vi "Font Style.vi"(2 "error in (no error)":errorcluster, 3 "Font Settings":T2={"Charset (-1)"=-1, "Weight (-1)"=-1, "Name"="", "Size"=" "}, 4 "Text Options":T1, 5 "NIReports.Report":refnum<k7>) -> (0 "error out":errorcluster, 1 "NIReports.Report out":refnum<k7>)   [LabVIEW 2015, in "NI_ReportGenerationCore.lvlib"]
uses:
  <vilib>/Utility/NIReport.llb/NI_ReportGenerationCore.lvlib
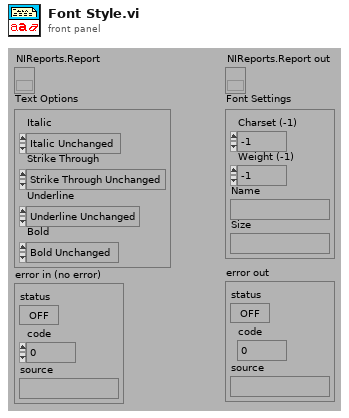
[diagram p1: front panel]
types:
  T1 = cluster{"Italic":enum16{"Italic Unchanged", "Italic On", "Italic Off"}, "Strike Through":enum16{"Strike Through Unchanged", "Strike Through On", "Strike Through Off"}, "Underline":enum16{"Underline Unchanged", "Underline On", "Underline Off"}, "Bold":enum16{"Bold Unchanged", "Bold On", "Bold Off"}}
  T2 = cluster{"Charset (-1)":i16, "Weight (-1)":i16, "Name":string, "Size":string}
  T3 = enum16{"Italic Unchanged", "Italic On", "Italic Off"}
  T4 = enum16{"Strike Through Unchanged", "Strike Through On", "Strike Through Off"}
  T5 = enum16{"Underline Unchanged", "Underline On", "Underline Off"}
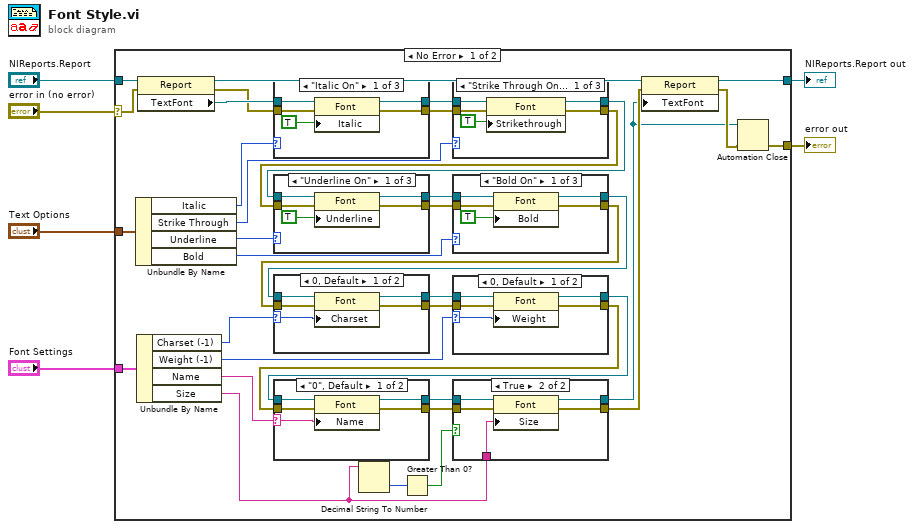
[diagram p0: block diagram]
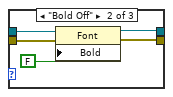
[diagram p6: hidden frame]
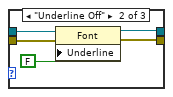
[diagram p8: hidden frame]
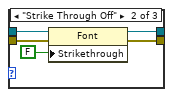
[diagram p10: hidden frame]
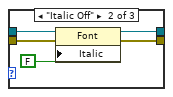
[diagram p12: hidden frame]
diagram:
  n1 = case shown="No Error" "error in (no error)" {
    selector: "error in (no error)" -> [w7 w119]
    tunnel: "Text Options" -> [w42 _]
    tunnel: "Font Settings" -> [w40 _]
    tunnel: "NIReports.Report" -> [w14 w120]
    tunnel: [w12 w120] -> w3
    tunnel: [w9 w119] -> w2
    frame No Error {
      n2 = Unbundle By Name(w42) -> ("Italic"=w41:T3, "Strike Through"=w35:T4, "Underline"=w32:T5, "Bold"=w29:enum16{"Bold Unchanged", "Bold On", "Bold Off"})
      n3 = Unbundle By Name(w40) -> ("Charset (-1)"=w28:i16, "Weight (-1)"=w23:i16, "Name"=w22:string, "Size"=w17:string)
      n4 = property class="Report"(reference=w14, error in=w7) -> (reference out=w13:refnum<k7>, error out=w38:errorcluster, "TextFont"=w39:refnum<k7>)
      n5 = case shown="\"Italic On\"" w41 {
        tunnel: w39 -> [w111 w115 w118]
        tunnel: w38 -> [w110 w114 w117]
        tunnel: [w108 w113 w118] -> w37
        tunnel: [w107 w112 w117] -> w36
        frame "Italic On" {
          n6 = property class="Font"(reference=w111, error in=w110, "Italic"=TRUE) -> (reference out=w108:refnum<k7>, error out=w107:errorcluster)
        }
        frame "Italic Off" {
          n7 = property class="Font"(reference=w115, error in=w114, "Italic"=FALSE) -> (reference out=w113:refnum<k7>, error out=w112:errorcluster)
        }
        frame "Italic Unchanged" {
        }
      }
      n8 = Decimal String To Number(string=w17) -> (number=w16:i32)  [unwired: 3 out]
      n9 = Greater Than 0?(x=w16) -> (x > 0?=w15:bool)
      n10 = case shown="\"Strike Through On\"" w35 {
        tunnel: w37 -> [w99 w103 w106]
        tunnel: w36 -> [w98 w102 w105]
        tunnel: [w96 w101 w106] -> w34
        tunnel: [w95 w100 w105] -> w33
        frame "Strike Through On" {
          n11 = property class="Font"(reference=w99, error in=w98, "Strikethrough"=TRUE ("Italic")) -> (reference out=w96:refnum<k7>, error out=w95:errorcluster)
        }
        frame "Strike Through Off" {
          n12 = property class="Font"(reference=w103, error in=w102, "Strikethrough"=FALSE ("Italic")) -> (reference out=w101:refnum<k7>, error out=w100:errorcluster)
        }
        frame "Strike Through Unchanged" {
        }
      }
      n13 = case shown="\"Underline On\"" w32 {
        tunnel: w34 -> [w87 w91 w94]
        tunnel: w33 -> [w86 w90 w93]
        tunnel: [w84 w89 w94] -> w30
        tunnel: [w83 w88 w93] -> w31
        frame "Underline On" {
          n14 = property class="Font"(reference=w87, error in=w86, "Underline"=TRUE ("Italic")) -> (reference out=w84:refnum<k7>, error out=w83:errorcluster)
        }
        frame "Underline Off" {
          n15 = property class="Font"(reference=w91, error in=w90, "Underline"=FALSE ("Italic")) -> (reference out=w89:refnum<k7>, error out=w88:errorcluster)
        }
        frame "Underline Unchanged" {
        }
      }
      n16 = case shown="\"Bold On\"" w29 {
        tunnel: w30 -> [w75 w79 w82]
        tunnel: w31 -> [w74 w78 w81]
        tunnel: [w72 w77 w82] -> w27
        tunnel: [w71 w76 w81] -> w26
        frame "Bold On" {
          n17 = property class="Font"(reference=w75, error in=w74, "Bold"=TRUE ("Italic")) -> (reference out=w72:refnum<k7>, error out=w71:errorcluster)
        }
        frame "Bold Off" {
          n18 = property class="Font"(reference=w79, error in=w78, "Bold"=FALSE ("Italic")) -> (reference out=w77:refnum<k7>, error out=w76:errorcluster)
        }
        frame "Bold Unchanged" {
        }
      }
      n19 = case shown="0, Default" w28 {
        selector: w28 -> [w66 _]
        tunnel: [w68 w70] -> w24
        tunnel: [w67 w69] -> w25
        tunnel: w27 -> [w65 w70]
        tunnel: w26 -> [w64 w69]
        frame 0, Default {
          n20 = property class="Font"(reference=w65, error in=w64, "Charset"=w66) -> (reference out=w68:refnum<k7>, error out=w67:errorcluster)
        }
        frame -1 {
        }
      }
      n21 = case shown="0, Default" w23 {
        selector: w23 -> [w59 _]
        tunnel: [w61 w63] -> w20
        tunnel: [w60 w62] -> w21
        tunnel: w24 -> [w58 w63]
        tunnel: w25 -> [w57 w62]
        frame 0, Default {
          n22 = property class="Font"(reference=w58, error in=w57, "Weight"=w59) -> (reference out=w61:refnum<k7>, error out=w60:errorcluster)
        }
        frame -1 {
        }
      }
      n23 = case shown="\"0\", Default" w22 {
        selector: w22 -> [w52 _]
        tunnel: [w54 w56] -> w19
        tunnel: [w53 w55] -> w18
        tunnel: w20 -> [w51 w56]
        tunnel: w21 -> [w50 w55]
        frame "0", Default {
          n24 = property class="Font"(reference=w51, error in=w50, "Name"=w52) -> (reference out=w54:refnum<k7>, error out=w53:errorcluster)
        }
        frame "" {
        }
      }
      n25 = case shown="True" w15 {
        tunnel: [w44 w49] -> w8
        tunnel: [w43 w48] -> w11
        tunnel: w19 -> [w44 w47]
        tunnel: w18 -> [w43 w46]
        tunnel: w17 -> [_ w45]
        frame False {
        }
        frame True {
          n26 = property class="Font"(reference=w47, error in=w46, "Size"=w45) -> (reference out=w49:refnum<k7>, error out=w48:errorcluster)
        }
      }
      n27 = property class="Report"(reference=w13, error in=w11, "TextFont"=w8) -> (reference out=w12:refnum<k7>, error out=w10:errorcluster)
      n28 = Automation Close(3:w10, 5:w8) -> (0:w9:errorcluster)
    }
    frame Error {
    }
  }
  "NIReports.Report out" <- w3
  "error out" <- w2
